vi "CoreComm.vi"(8 "error in (no error)":errorcluster, 9 "Data":variant, 10 "Msg":T1, 11 "Module in":refnum<class "Module.lvclass">) -> (0 "error out":errorcluster, 3 "Module out":refnum<class "Module.lvclass">)   [LabVIEW 2025, in "Module.lvlib" / "Module.lvclass"]
uses:
  Module.lvclass
  Msg.ctl
  Msg&Data.ctl
  Module.lvclass/Module.ctl
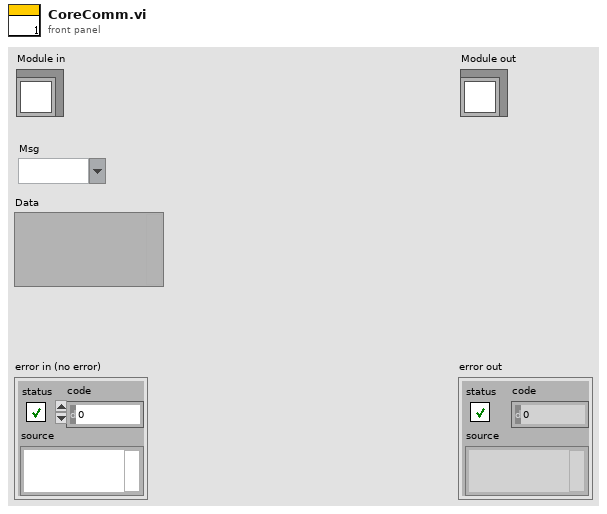
[diagram p1: front panel]
types:
  T1 = typedef "Msg.ctl" = string
  T2 = typedef "Msg&Data.ctl" = cluster{"Msg":T1, "Data":variant}
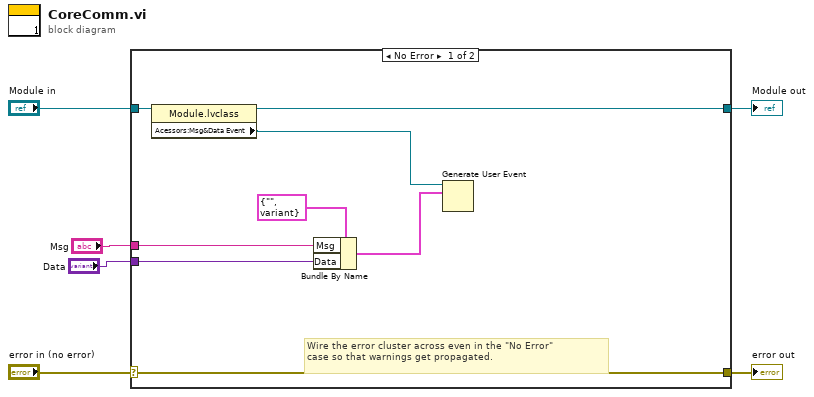
[diagram p0: block diagram]
diagram:
  n1 = case shown="No Error" "error in (no error)" {
    selector: "error in (no error)" -> [w13 w16]
    tunnel: [w13 w16] -> w5
    tunnel: [w12 w15] -> w3
    tunnel: "Module in" -> [w14 w15]
    tunnel: "Msg" -> [w8 _]
    tunnel: "Data" -> [w7 _]
    frame No Error {
      # "Wire the error cluster across even in the \"No Error\"\ncase so that warnings get propagated."
      n2 = property class="Module.lvclass"(reference=w14) -> (reference out=w12:refnum<class "Module.lvclass">, "Acessors:Msg&Data Event"=w9:refnum<user-event>)  [unwired: 1 in, 1 out]
      n3 = Bundle By Name(cluster=T2 {"Msg"="", "Data"=variant} ("Msg&Data"), "Msg"=w8, "Data"=w7) -> (w11:T2)
      n4 = Generate User Event(user event=w9, event data cluster=w11) -> ()  [unwired: 2 in, 2 out]
    }
    frame Error {
    }
  }
  "error out" <- w5
  "Module out" <- w3
